vi "Prepare Response.vi"(8 "error in (no error)":errorcluster, 11 "UNSUBSCRIBE in":refnum<class "UNSUBSCRIBE.lvclass">) -> (0 "error out":errorcluster, 1 "response prepared?":bool, 2 "ControlPacket response":refnum<class "ControlPacket.lvclass">, 3 "UNSUBSCRIBE out":refnum<class "UNSUBSCRIBE.lvclass">)   [LabVIEW 2013, in "MQTT_Control_Packets.lvlib" / "UNSUBSCRIBE.lvclass"]
uses:
  UNSUBSCRIBE.lvclass
  ControlPacket/ControlPacket.lvclass
  ControlPacket/ControlPacket.lvclass/ControlPacket.ctl
  UNSUBACK/UNSUBACK.lvclass
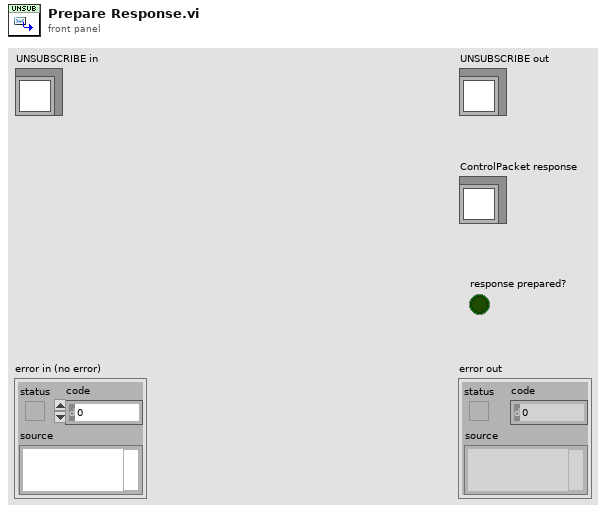
[diagram p1: front panel]
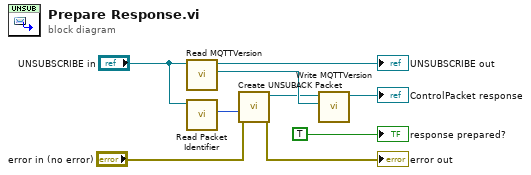
[diagram p0: block diagram]
diagram:
  n1 = call "Read MQTTVersion.vi"("ControlPacket in"="UNSUBSCRIBE in") -> ("MQTTVersion"=w9:refnum<class "MQTTVersion.lvclass">, "ControlPacket out"=→"UNSUBSCRIBE out":refnum<class "UNSUBSCRIBE.lvclass">)  [unwired: 9 in]
  n2 = call "Read Packet Identifier.vi"("ControlPacket in"="UNSUBSCRIBE in") -> ("Packet Identifier"=w3:u16)  [unwired: 9 in, 1 out]
  n3 = call "Create UNSUBACK Packet.vi"("error in (no error)"="error in (no error)", "Packet ID"=w3) -> ("error out"=→"error out":errorcluster, "UNSUBACK out"=w8:refnum<class "UNSUBACK.lvclass">)  [unwired: 7 in, 1 out]
  n4 = call "Write MQTTVersion.vi"("MQTTVersion"=w9, "ControlPacket in"=w8) -> ("ControlPacket out"=→"ControlPacket response":refnum<class "UNSUBACK.lvclass">)  [unwired: 9 in]
  "response prepared?" <- TRUE ("response prepared?")
